vi "voltage.vi"(11 "Qube":refnum<class "System.lvclass">) -> (3 "Qube":refnum<class "System.lvclass">)   [LabVIEW 2021, in "System.lvclass"]
uses:
  System.lvclass
  System.lvclass/System.ctl
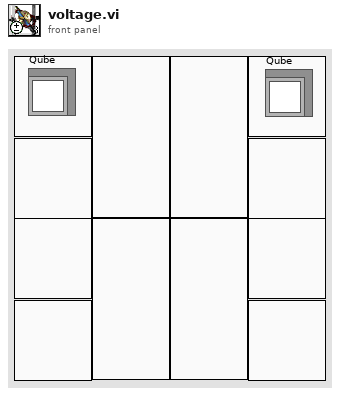
[diagram p1: front panel]
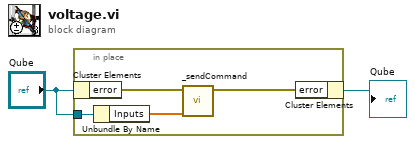
[diagram p0: block diagram]
diagram:
  n1 = in-place {
    in-place-border: "Qube" -> [w3]
    n2 = in-place-cluster #1("Qube") -> ("error"=w6:errorcluster)
    n3 = Unbundle By Name(w3) -> ("Inputs"=w4:dbl[])
    n4 = call "_sendCommand.vi"("FBLR"=w4, "error in (no error)"=w6) -> ("error out"=w5:errorcluster)  [unwired: 9 in]
    n5 = in-place-cluster #1("error"=w5) -> (→"Qube":refnum<class "System.lvclass">)
  }
